vi "CC.vi"(1 "测试温度":dbl, 5 "簇 2":T1, 6 "Scanning Mode":u16(ring)=1 items=["Linear", "Log"], 7 "开始频率":dbl[](array[numeric])=[20.0, 5000000.0, 100.0], 8 "error in (no error)":errorcluster caption="错误输入（无错误）", 9 "簇":T2={"电容计地址"="USB0::0x0471::0x2826::QF71600867::INSTR", "高温地址"="USB0::0x0471::0x2826::QF71600867::INSTR", "高温地址 2"="USB0::0x0471::0x2826::QF71600867::INSTR"}, 10 "文本":path, 11 "表格":path) -> (0 "错误输出":cluster{"状态":bool, "代码":i32, "源":string})   [LabVIEW 2017]
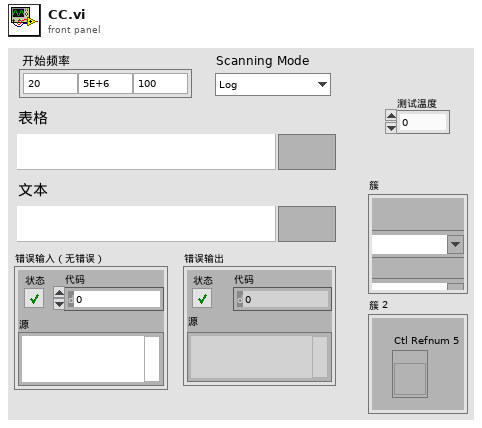
[diagram p1: front panel]
types:
  T1 = cluster{"Ctl Refnum":refnum<vi>, "Ctl Refnum 2":refnum<vi>, "Ctl Refnum 3":refnum<vi>, "Ctl Refnum 4":refnum<vi>, "Ctl Refnum 5":refnum<vi>}
  T2 = cluster{"电容计地址":refnum<visa-resource-name>, "高温地址":refnum<visa-resource-name>, "高温地址 2":refnum<visa-resource-name>}
  T3 = enum16{"open", "replace", "create", "open or create", "replace or create", "replace or create with confirmation"}
  T4 = cluster{"高温地址":refnum<visa-resource-name>, "高温地址 2":refnum<visa-resource-name>}
  T5 = cluster{"Array":string[][], "error out":errorcluster}
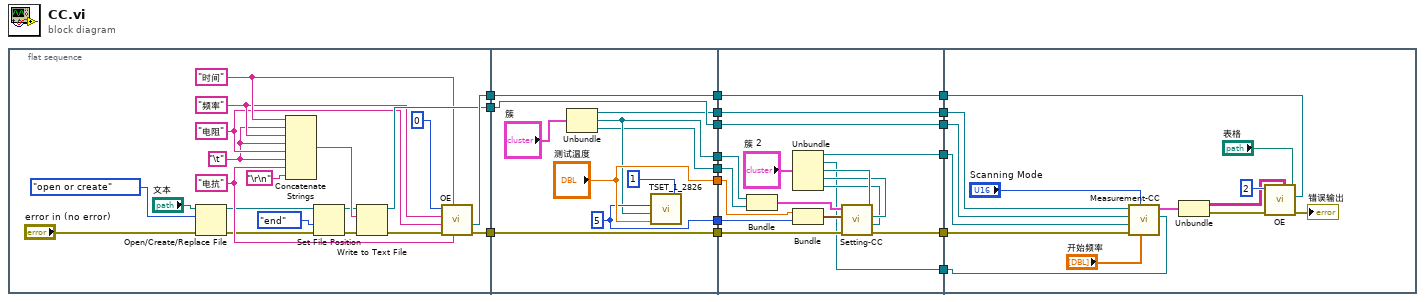
[diagram p0: block diagram]
diagram:
  n1 = flat-sequence {
    tunnel: [w34] -> w17
    tunnel: [w29] -> w16
    tunnel: [w33] -> w15
    tunnel: w17 -> [w47]
    tunnel: [w47] -> w14
    tunnel: w16 -> [w46]
    tunnel: [w46] -> w12
    tunnel: w15 -> [w45]
    tunnel: [w45] -> w10
    tunnel: [w40] -> w8
    tunnel: ["测试温度"] -> w7
    tunnel: [w42] -> w6
    tunnel: [w39] -> w5
    tunnel: [w38] -> w3
    tunnel: w14 -> [w57]
    tunnel: [w56] -> w13
    tunnel: w12 -> [w64]
    tunnel: [w64] -> w11
    tunnel: w10 -> [w63]
    tunnel: [w63] -> w9
    tunnel: w8 -> [w59]
    tunnel: w7 -> [w62]
    tunnel: w6 -> [w61]
    tunnel: w5 -> [w55]
    tunnel: [w54] -> w4
    tunnel: w3 -> [w54]
    tunnel: [w49] -> w2
    tunnel: [w48] -> w1
    tunnel: w13 -> [w78]
    tunnel: w11 -> [w68]
    tunnel: w9 -> [w75]
    tunnel: w4 -> [w67]
    tunnel: w2 -> [w66]
    tunnel: w1 -> [w65]
    frame #0 {
      w24 = "电抗" ("字符串")
      w26 = "电阻" ("字符串")
      w27 = "频率" ("字符串")
      w25 = "\t"
      w28 = "时间" ("字符串")
      n2 = Open/Create/Replace File(file path (use dialog)="文本", error in="error in (no error)", operation (0:open)=T3."open or create" ("操作(0:open)")) -> (refnum out=w21:refnum<file>, error out=w19:errorcluster)  [unwired: 4 out]
      n3 = Concatenate Strings(w28, w25, w27, w25, w26, w25, w24, "\r\n") -> (w22:string)
      n4 = Set File Position(refnum=w21, from (0:start)=enum16{"start", "end", "current"}."end" ("自（0:起始）"), error in=w19) -> (refnum out=w20:refnum<file>, error out=w18:errorcluster)  [unwired: 1 out]
      n5 = Write to Text File(file (use dialog)=w20, text=w22, error in=w18) -> (refnum out=w29:refnum<file>, error out=w30:errorcluster)  [unwired: 2 out]
      n6 = call "OE.vi"("String 4"=w24, "String"=w28, "error in (no error)"=w30, "String 3"=w26, "String 2"=w27, "Numeric"=0) -> ("error out"=w34:errorcluster, "report out"=w33:refnum<class "NI_report.lvclass">)  [unwired: 3 in, 1 out]
    }
    frame #1 {
      w42 = 5
      n7 = Unbundle("簇") -> ("电容计地址"=w38:refnum<visa-resource-name>, "高温地址"=w40:refnum<visa-resource-name>, "高温地址 2"=w39:refnum<visa-resource-name>)
      n8 = call "TSET_1_2826.vi"("Address No."=i8 1, "T-Ending, C"="测试温度", "VISA resource name"=w40, "cooling/heating rate, C/min"=w42) -> ()  [unwired: 1 in]
    }
    frame #2 {
      n9 = Bundle("高温地址"=w59, "高温地址 2"=w55) -> (w58:T4)  [unwired: 1 in]
      n10 = Unbundle("簇 2") -> ("Ctl Refnum"=w49:refnum<vi>, "Ctl Refnum 2"=w48:refnum<vi>, "Ctl Refnum 3"=w52:refnum<vi>, "Ctl Refnum 4"=w51:refnum<vi>, "Ctl Refnum 5"=w50:refnum<vi>)
      n11 = Bundle("测试温度"=w62, w61) -> (w60:cluster{"测试温度":dbl, i32})  [unwired: 1 in]
      n12 = call "Setting-CC.vi"("Ctl引用句柄 3"=w50, "Ctl引用句柄 2"=w51, "Ctl引用句柄"=w52, "error in (no error)"=w57, "Cluster 2"=w60, "Cluster"=w58) -> ("error out"=w56:errorcluster)  [unwired: 5 in]
    }
    frame #3 {
      n13 = call "Measurement-CC.vi"("Ctl Refnum 2"=w65, "开始频率"="开始频率", "Scanning Mode"="Scanning Mode", "error in (no error)"=w78, "Ctl Refnum"=w66, "BSFR"=w68, "电阻地址"=w67) -> ("Cluster"=w71:T5)  [unwired: 4 in]
      n14 = Unbundle(w71) -> ("Array"=w73:string[][], "error out"=w72:errorcluster)
      n15 = call "OE.vi"("report in"=w75, "表格数据路径："="表格", "Array"=w73, "error in (no error)"=w72, "Numeric"=2) -> ("error out"=→"错误输出":errorcluster)  [unwired: 4 in, 2 out]
    }
  }
